vi "task_1.vi"(8 "Input 2":dbl, 9 "Input 1":dbl) -> (0 "Output 2":dbl format="%#_13g", 1 "Output 1":dbl format="%#_13g")   [LabVIEW 2023]
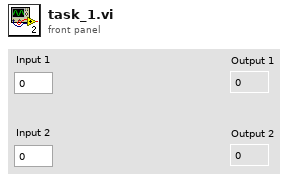
[diagram p1: front panel]
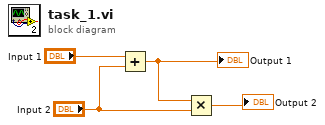
[diagram p0: block diagram]
diagram:
  n1 = Add(x="Input 1", y="Input 2") -> (x+y=w2:dbl)
  "Output 1" <- w2
  n2 = Multiply(x=w2, y="Input 2") -> (x*y=→"Output 2":dbl)
